vi "CODCr插入数据.vi"(1 "data":T4 {"单位" items=["ug/L", "mg/L", "ppm", "mg/m3", "cm", "ppb", "ug/m3", "%", "nmol/mol", "umol/mol", "MPN/L", "MPN/100ml", "ng/m3", "NTU", "无量纲", "ms/cm", "us/cm"]}, 7 "测量模式":T3(ring)=enum."水样测试", 9 "数据类型":T2=enum."M", 11 "error in (no error)":errorcluster) -> (15 "error out":errorcluster)   [LabVIEW 2016, in "CODCr库.lvlib"]
uses:
  <vilib>/Utility/error.llb/DialogType.ctl
panel:
  out "data输出":T1
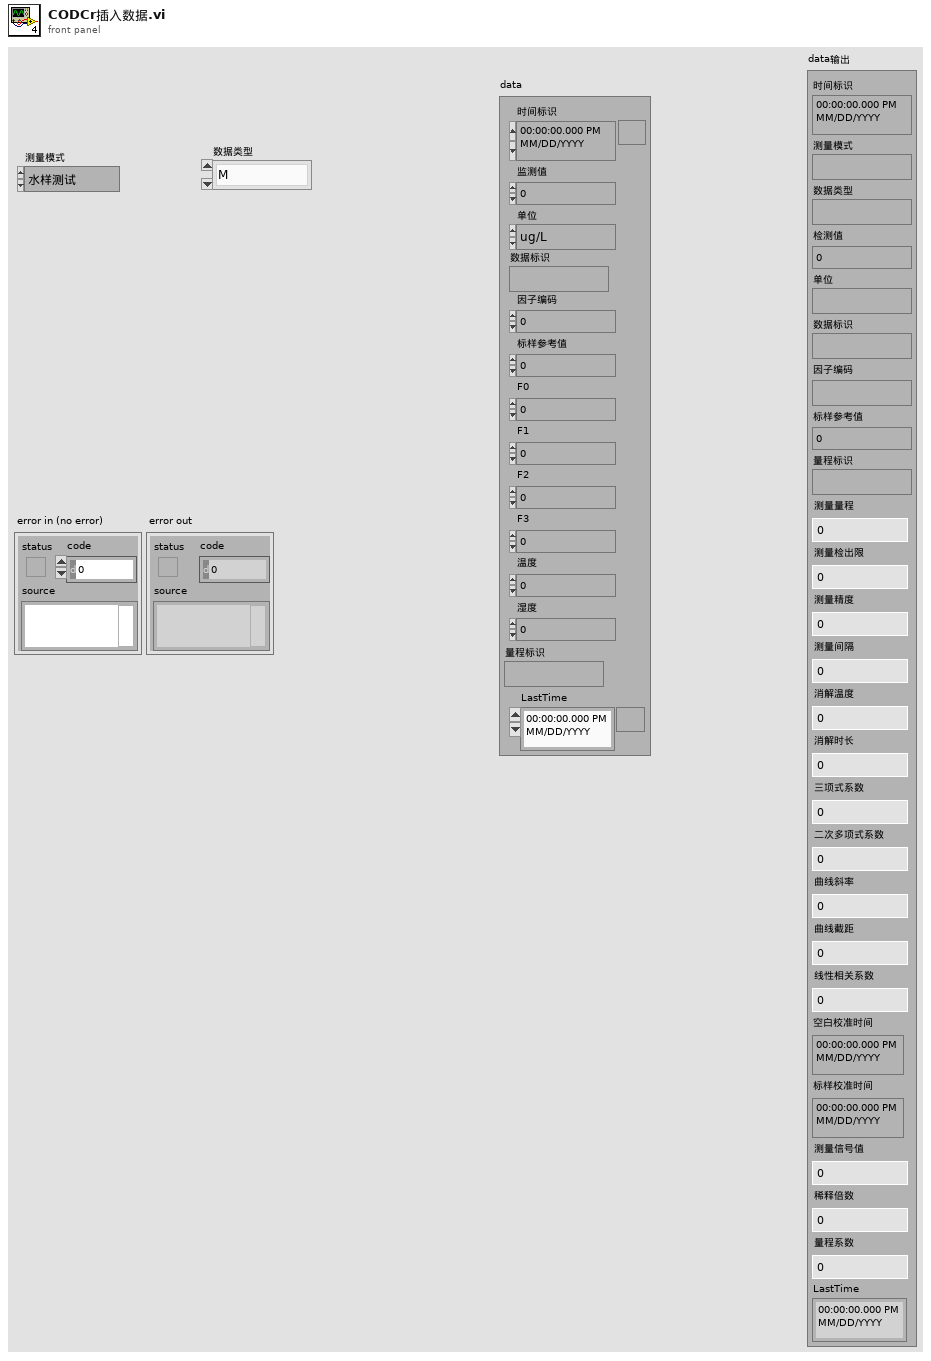
[diagram p1: front panel]
types:
  T1 = cluster{"时间标识":timestamp, "测量模式":string, "数据类型":string, "检测值":sgl, "单位":string, "数据标识":string, "因子编码":string, "标样参考值":sgl, "量程标识":string, "测量量程":sgl, "测量检出限":sgl, "测量精度":sgl, "测量间隔":sgl, "消解温度":sgl, "消解时长":sgl, "三项式系数":sgl, "二次多项式系数":sgl, "曲线斜率":sgl, "曲线截距":sgl, "线性相关系数":sgl, "空白校准时间":timestamp, "标样校准时间":timestamp, "测量信号值":sgl, "稀释倍数":sgl, "量程系数":sgl, "LastTime":timestamp}
  T2 = typedef "测试模式.ctl" = enum16{"N", "M", "P"}
  T3 = enum16{"空闲", "水样测试", "标样核查", "零点核查", "跨度核查", "空白测试", "平行样测试", "加标回收", "空白校准", "标样校准", "初始化（清洗）"}
  T4 = cluster{"时间标识":timestamp, "监测值":sgl, "单位":u16, "数据标识":string, "因子编码":u32, "标样参考值":sgl, "F0":sgl, "F1":sgl, "F2":sgl, "F3":sgl, "温度":sgl, "湿度":sgl, "量程标识":string, "LastTime":timestamp}
  T5 = typedef "DialogType.ctl" = u16
  T6 = cluster{"测量量程":dbl, "测量精度":dbl, "测量间隔":dbl, "消解温度":dbl, "消解时长":dbl, "空白校准时间":timestamp, "曲线截距":dbl, "曲线斜率":dbl, "测量检出限":dbl, "测量信号值":dbl, "线性相关系数":dbl, "二次多项式系数":dbl, "标样校准时间":timestamp, "稀释倍数":dbl, "三项式系数":dbl, "空白标定系数":dbl, "量程系数":dbl}
  T7 = cluster{"时间标识":timestamp, "测量模式":string, "数据类型":string, "检测值":sgl, "单位":string, "数据标识":string, "因子编码":string, "标样参考值":sgl, "量程标识":string, "LastTime":timestamp}
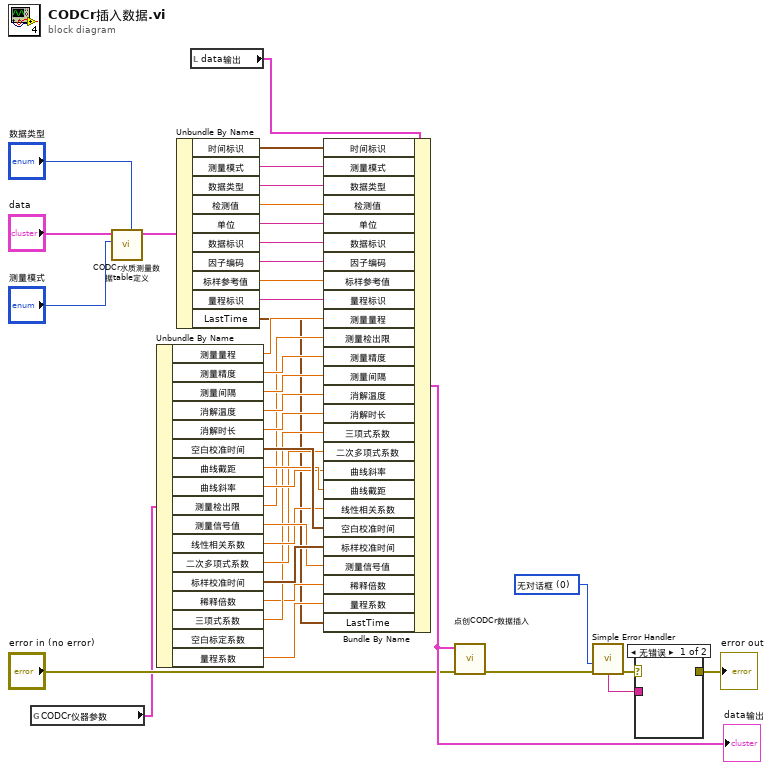
[diagram p0: block diagram]
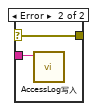
[diagram p2: hidden frame]
diagram:
  w38 = T5 0 items=["无对话框", "确定信息", "继续或停止信息", "确定信息＋警告", "继续/停止+警告"] ("type of dialog (OK msg:1)")
  n1 = global read "CODcr全局变量.vi" "CODCr仪器参数"() -> (w27:T6)
  n2 = call "CODCr水质测量数据table定义.vi"("数据类型"="数据类型", "测量模式"="测量模式", "data"="data") -> ("data输出"=w28:T7)  [unwired: 6 in, 2 out]
  n3 = Unbundle By Name(w27) -> ("测量量程"=w26:dbl, "测量精度"=w25:dbl, "测量间隔"=w24:dbl, "消解温度"=w23:dbl, "消解时长"=w22:dbl, "空白校准时间"=w21:timestamp, "曲线截距"=w19:dbl, "曲线斜率"=w18:dbl, "测量检出限"=w17:dbl, "测量信号值"=w16:dbl, "线性相关系数"=w15:dbl, "二次多项式系数"=w14:dbl, "标样校准时间"=w20:timestamp, "稀释倍数"=w12:dbl, "三项式系数"=w13:dbl, "量程系数"=w11:dbl)  [unwired: 1 out]
  n4 = Unbundle By Name(w28) -> ("时间标识"=w1:timestamp, "测量模式"=w2:string, "数据类型"=w3:string, "检测值"=w4:sgl, "单位"=w5:string, "数据标识"=w6:string, "因子编码"=w7:string, "标样参考值"=w8:sgl, "量程标识"=w9:string, "LastTime"=w10:timestamp)
  n5 = local read "data输出"() -> (w34:T1)
  n6 = Bundle By Name(cluster=w34, "时间标识"=w1, "测量模式"=w2, "数据类型"=w3, "检测值"=w4, "单位"=w5, "数据标识"=w6, "因子编码"=w7, "标样参考值"=w8, "量程标识"=w9, "测量量程"=w26, "测量检出限"=w17, "测量精度"=w25, "测量间隔"=w24, "消解温度"=w23, "消解时长"=w22, "三项式系数"=w13, "二次多项式系数"=w14, "曲线斜率"=w18, "曲线截距"=w19, "线性相关系数"=w15, "空白校准时间"=w21, "标样校准时间"=w20, "测量信号值"=w16, "稀释倍数"=w12, "量程系数"=w11, "LastTime"=w10) -> (w30:T1)
  "data输出" <- w30
  n7 = call "点创CODCr数据插入.vi"("data输出"=w30, "错误输入（无错误）"="error in (no error)") -> ("错误输出"=w31:errorcluster)  [unwired: 8 in]
  n8 = call <vilib>:"Simple Error Handler.vi"("type of dialog (OK msg:1)"=w38, "error in (no error)"=w31) -> ("error out"=w37:errorcluster, "message"=w36:string)  [unwired: 3 in, 3 out]
  n9 = case shown="无错误" w37 {
    selector: w37 -> [_ w40]
    tunnel: [_ w40] -> w35
    tunnel: w36 -> [_ w41]
    frame No Error {
    }
    frame Error {
      n10 = call "AccessLog写入.vi"("Log"=w41) -> ()  [unwired: 11 in]
    }
  }
  "error out" <- w35
